vi "Drive Encoder Test v3.vi"   [LabVIEW 2014]
uses:
  <vilib>/Rock Robotics/WPI/DriverStation/WPI_DriverStationRobotMode2.ctl
  Begin/Global Variables.vi
  Begin/Global RefNums.vi
  Begin/Global Constants.vi
  <vilib>/Utility/file.llb/Write To Spreadsheet File (DBL).vi
types:
  T1 = typedef "WPI_DriverStationRobotMode2.ctl" = enum16{"Autonomous Disabled", "Autonomous Enabled", "Teleop Disabled", "Teleop Enabled", "Disconnected", "Finish", "Test Disabled", "Test Enabled", "Emergency Stopped"}
  T2 = typedef "WPI_AnalogChannelDevRef.ctl" = cluster{"DevStatus":errorcluster, "Controller":T3, "Analog Channel":T4}
  T3 = typedef "FPGA_TypedefAnalogModule.ctl" = enum16{"Controller 1"}
  T4 = typedef "FPGA_AIChannel.ctl" = enum8{"AI 0", "AI 1", "AI 2", "AI 3", "AI MXP 0", "AI MXP 1", "AI MXP 2", "AI MXP 3", "Invalid"}
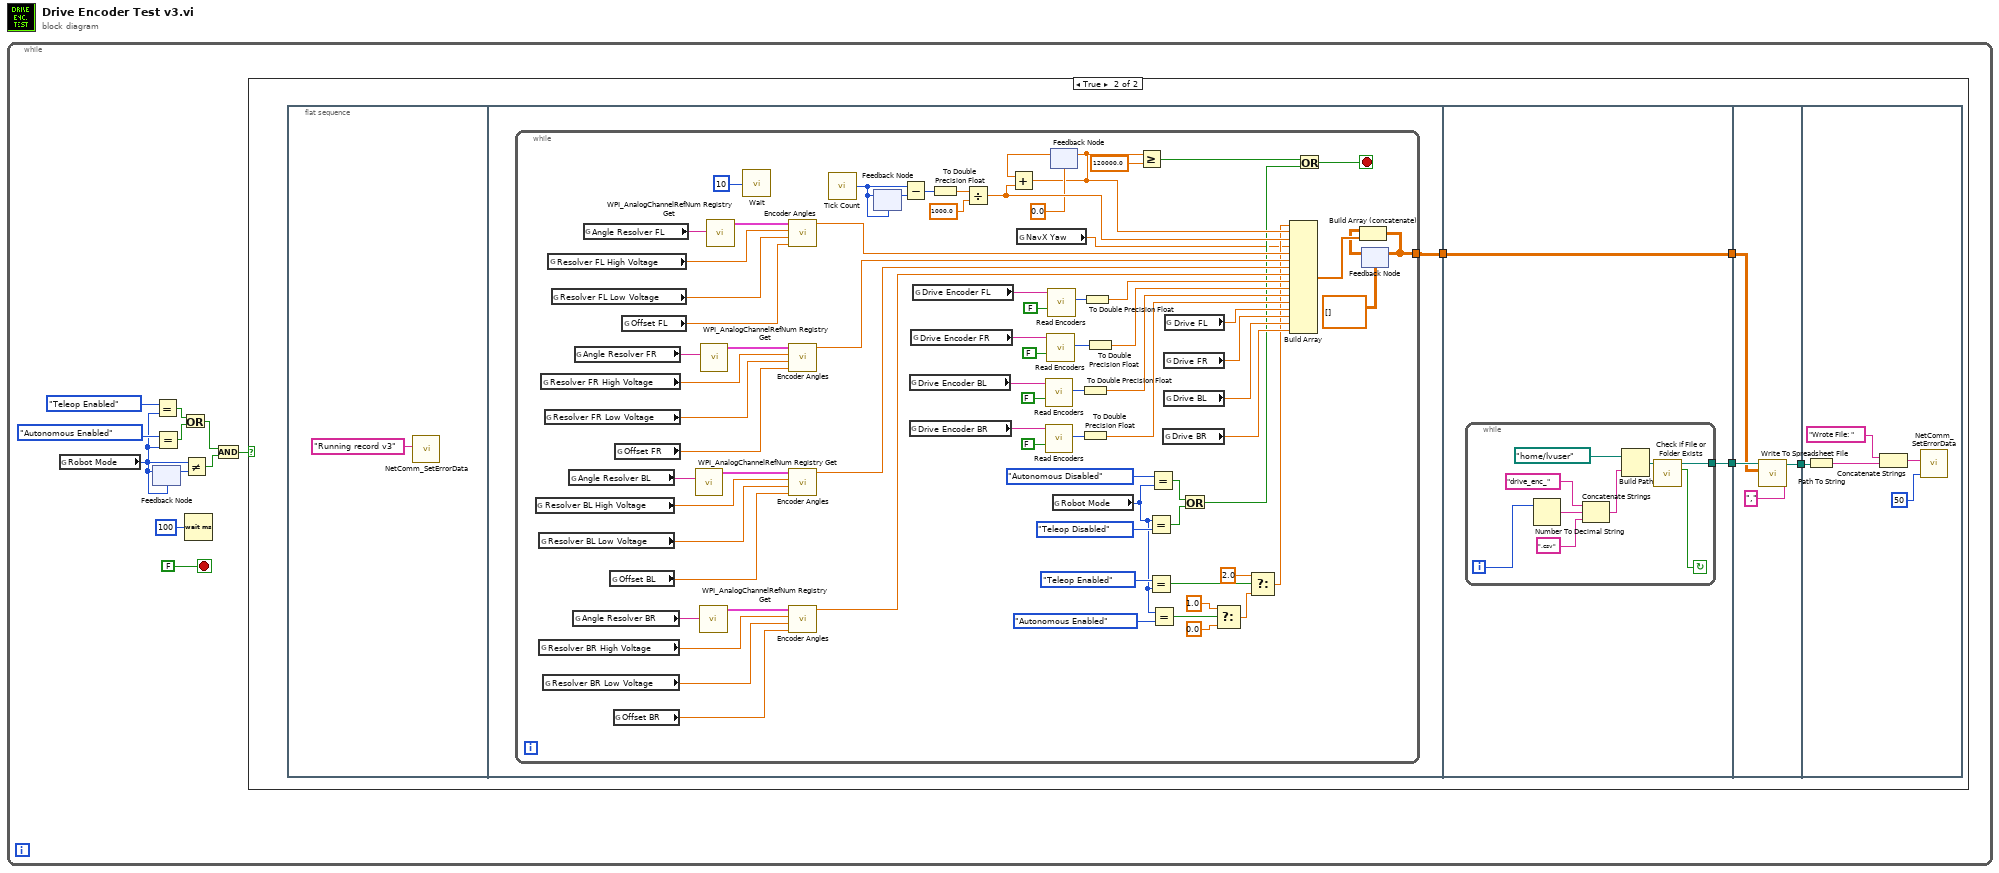
[diagram p0: block diagram]
diagram:
  n1 = while {
    stop <- FALSE stop-if-true
    n2 = global read "Global Variables.vi" "Robot Mode"() -> (w5:T1)
    n3 = feedback-in #1(w5) -> ()
    n4 = feedback #1(w5) -> (w9:T1)
    n5 = Equal?(x=WPI_DriverStationRobotMode2."Teleop Enabled", y=w5) -> (x = y?=w4:bool)
    n6 = Equal?(x=WPI_DriverStationRobotMode2."Autonomous Enabled", y=w5) -> (x = y?=w3:bool)
    n7 = Or(x=w4, y=w3) -> (x .or. y?=w2:bool)
    n8 = Not Equal?(x=w5, y=w9) -> (x != y?=w8:bool)
    n9 = Wait (ms)(milliseconds to wait=u32 100) -> ()  [unwired: 1 out]
    n10 = And(x=w2, y=w8) -> (x .and. y?=w1:bool)
    n11 = case shown="True" w1 {
      frame False {
      }
      frame True {
        n12 = flat-sequence {
          tunnel: [w17] -> w15
          tunnel: w15 -> [w95]
          tunnel: [w96] -> w14
          tunnel: [w95] -> w13
          tunnel: w14 -> [w108]
          tunnel: w13 -> [w107]
          tunnel: [w106] -> w12
          tunnel: w12 -> [w110]
          frame #0 {
            n13 = call <vilib>:"NetComm_SetErrorData.vi"("Error Data"="Running record v3") -> ()  [unwired: 3 in, 8 out]
          }
          frame #1 {
            n14 = while {
              tunnel: [w55] -> w17
              stop <- w18 stop-if-true
              n15 = global read "Global Constants.vi" "Resolver BL High Voltage"() -> (w80:dbl)
              n16 = global read "Global Constants.vi" "Resolver BL Low Voltage"() -> (w79:dbl)
              n17 = global read "Global Constants.vi" "Resolver BR High Voltage"() -> (w82:dbl)
              n18 = global read "Global Constants.vi" "Resolver FR High Voltage"() -> (w86:dbl)
              n19 = global read "Global Constants.vi" "Resolver BR Low Voltage"() -> (w81:dbl)
              n20 = global read "Global Constants.vi" "Resolver FR Low Voltage"() -> (w85:dbl)
              n21 = global read "Global Constants.vi" "Resolver FL High Voltage"() -> (w84:dbl)
              n22 = global read "Global Constants.vi" "Resolver FL Low Voltage"() -> (w83:dbl)
              n23 = global read "Global RefNums.vi" "Angle Resolver BL"() -> (w93:string)
              n24 = global read "Global RefNums.vi" "Angle Resolver BR"() -> (w92:string)
              n25 = global read "Global RefNums.vi" "Angle Resolver FR"() -> (w94:string)
              n26 = global read "Global RefNums.vi" "Angle Resolver FL"() -> (w91:string)
              n27 = global read "Global Constants.vi" "Offset BL"() -> (w75:dbl)
              n28 = global read "Global Constants.vi" "Offset BR"() -> (w76:dbl)
              n29 = global read "Global Constants.vi" "Offset FR"() -> (w78:dbl)
              n30 = global read "Global Constants.vi" "Offset FL"() -> (w77:dbl)
              n31 = call <vilib>:"WPI_AnalogChannelRefNum Registry Get.vi"("refnum name"=w93) -> ("AIDeviceRef"=w87:T2)  [unwired: 9 in, 1 out]
              n32 = call <vilib>:"WPI_AnalogChannelRefNum Registry Get.vi"("refnum name"=w92) -> ("AIDeviceRef"=w88:T2)  [unwired: 9 in, 1 out]
              n33 = call <vilib>:"WPI_AnalogChannelRefNum Registry Get.vi"("refnum name"=w94) -> ("AIDeviceRef"=w90:T2)  [unwired: 9 in, 1 out]
              n34 = call <vilib>:"WPI_AnalogChannelRefNum Registry Get.vi"("refnum name"=w91) -> ("AIDeviceRef"=w89:T2)  [unwired: 9 in, 1 out]
              n35 = call "Wait"("Count(mSec)"=u32 10) -> ()  [unwired: 1 out]
              n36 = call "Encoder Angles.vi"("calibration angle"=w77, "low voltage"=w83, "top voltage"=w84, "AIDeviceRef Encoder"=w89) -> ("encoder angle"=w47:dbl)  [unwired: 7 in]
              n37 = call "Encoder Angles.vi"("calibration angle"=w78, "low voltage"=w85, "top voltage"=w86, "AIDeviceRef Encoder"=w90) -> ("encoder angle"=w46:dbl)  [unwired: 7 in]
              n38 = call "Encoder Angles.vi"("calibration angle"=w75, "low voltage"=w79, "top voltage"=w80, "AIDeviceRef Encoder"=w87) -> ("encoder angle"=w45:dbl)  [unwired: 7 in]
              n39 = call "Encoder Angles.vi"("calibration angle"=w76, "low voltage"=w81, "top voltage"=w82, "AIDeviceRef Encoder"=w88) -> ("encoder angle"=w44:dbl)  [unwired: 7 in]
              n40 = call "Tick Count"() -> ("Tick Count(uSec)"=w62:u32)
              n41 = feedback-in #2(w62) -> ()
              n42 = feedback #2(w62) -> (w61:u32)
              n43 = Subtract(x=w62, y=w61) -> (x-y=w53:u32)
              n44 = global read "Global RefNums.vi" "Drive Encoder BL"() -> (w74:string)
              n45 = global read "Global RefNums.vi" "Drive Encoder BR"() -> (w71:string)
              n46 = global read "Global RefNums.vi" "Drive Encoder FR"() -> (w69:string)
              n47 = global read "Global RefNums.vi" "Drive Encoder FL"() -> (w70:string)
              n48 = To Double Precision Float(number=w53) -> (double precision float=w60:dbl)
              n49 = Divide(x=w60, y=1000.0) -> (x/y=w52:dbl)
              n50 = global read "Global Variables.vi" "NavX Yaw"() -> (w20:dbl)
              n51 = call "Read Encoders.vi"("Reset Encoders"=FALSE, "Encoder"=w74) -> ("Counts"=w66:i32)  [unwired: 9 in]
              n52 = call "Read Encoders.vi"("Reset Encoders"=FALSE, "Encoder"=w71) -> ("Counts"=w63:i32)  [unwired: 9 in]
              n53 = call "Read Encoders.vi"("Reset Encoders"=FALSE, "Encoder"=w69) -> ("Counts"=w65:i32)  [unwired: 9 in]
              n54 = call "Read Encoders.vi"("Reset Encoders"=FALSE, "Encoder"=w70) -> ("Counts"=w64:i32)  [unwired: 9 in]
              n55 = feedback #3(0.0) -> (w51:dbl)
              n56 = Add(x=w51, y=w52) -> (x+y=w48:dbl)
              n57 = feedback-in #3(w48) -> ()
              n58 = global read "Global Variables.vi" "Robot Mode"() -> (w27:T1)
              n59 = To Double Precision Float(number=w66) -> (double precision float=w41:dbl)
              n60 = To Double Precision Float(number=w63) -> (double precision float=w40:dbl)
              n61 = To Double Precision Float(number=w64) -> (double precision float=w43:dbl)
              n62 = To Double Precision Float(number=w65) -> (double precision float=w42:dbl)
              n63 = Greater Or Equal?(x=w48, y=120000.0) -> (x >= y?=w19:bool)
              n64 = Equal?(x=w27, y=WPI_DriverStationRobotMode2."Teleop Disabled" ("x")) -> (x = y?=w33:bool)
              n65 = Equal?(x=WPI_DriverStationRobotMode2."Teleop Enabled", y=w27) -> (x = y?=w29:bool)
              n66 = Equal?(x=WPI_DriverStationRobotMode2."Autonomous Disabled", y=w27) -> (x = y?=w32:bool)
              n67 = Equal?(x=w27, y=WPI_DriverStationRobotMode2."Autonomous Enabled" ("x")) -> (x = y?=w26:bool)
              n68 = global read "Global Variables.vi" "Drive BR"() -> (w36:dbl)
              n69 = global read "Global Variables.vi" "Drive FR"() -> (w38:dbl)
              n70 = global read "Global Variables.vi" "Drive BL"() -> (w37:dbl)
              n71 = global read "Global Variables.vi" "Drive FL"() -> (w39:dbl)
              n72 = Or(x=w32, y=w33) -> (x .or. y?=w31:bool)
              n73 = Select(t=1.0, s=w26, f=0.0) -> (s? t:f=w25:dbl)
              n74 = Select(t=2.0, s=w29, f=w25) -> (s? t:f=w21:dbl)
              n75 = Build Array(w21, w48, w52, w20, w47, w46, w45, w44, w43, w42, w41, w40, w39, w38, w37, w36) -> (w58:dbl[])
              n76 = Or(x=w19, y=w31) -> (x .or. y?=w18:bool)
              n77 = feedback #4(dbl[][] []) -> (w57:dbl[][])
              n78 = Build Array (concatenate)(w57, w58) -> (w55:dbl[][])
              n79 = feedback-in #4(w55) -> ()
            }
          }
          frame #2 {
            n80 = while {
              tunnel: [w98] -> w96
              i -> [w97]
              stop <- w105 continue-if-true
              n81 = Number To Decimal String(number=w97) -> (decimal integer string=w102:string)  [unwired: 1 in]
              n82 = Concatenate Strings("drive_enc_", w102, ".csv") -> (w101:string)
              n83 = Build Path(base path=path "/home/lvuser" ("file path (dialog if empty)"), name or relative path=w101) -> (appended path=w104:path)
              n84 = call <vilib>:"Check if File or Folder Exists.vi"("path"=w104) -> ("file or folder exists?"=w105:bool, "dup path"=w98:path)  [unwired: 8 in, 1 out]
            }
          }
          frame #3 {
            n85 = call-poly <vilib>:"Write To Spreadsheet File.vi"("delimiter (\\t)"="," ("delimiter (\\t)"), "2D data"=w107, "file path (dialog if empty)"=w108) -> ("new file path (Not A Path if cancelled)"=w106:path)  [unwired: 5 in]
          }
          frame #4 {
            n86 = Path To String(path=w110) -> (string=w114:string)
            n87 = Concatenate Strings("Wrote File: ", w114) -> (w112:string)
            n88 = call <vilib>:"NetComm_SetErrorData.vi"("Timeout (ms)"=50, "Error Data"=w112) -> ()  [unwired: 2 in, 8 out]
          }
        }
      }
    }
  }
